vi "Populate VI Help.vi"(5 "API Dir":path[](array[path]), 6 "options":cluster{"Force?(F)":bool, "Show FP":bool}={"Force?(F)"=FALSE, "Show FP"=TRUE}, 7 "doc dir":path, 8 "error in (no error)":errorcluster, 10 "Language Ring":string(combo)="English(en-us)") -> (0 "error out":errorcluster)   [LabVIEW 2017, in "csmdoc.lvlib"]
uses:
  csmdoc.lvlib
  _Typedef/DocElement.ctl
  _Shared/CSM Shared.lvlib
  _tool/_batchEditorDialog/batchEditorDialog.lvlib
  Communicable State Machine.lvlib
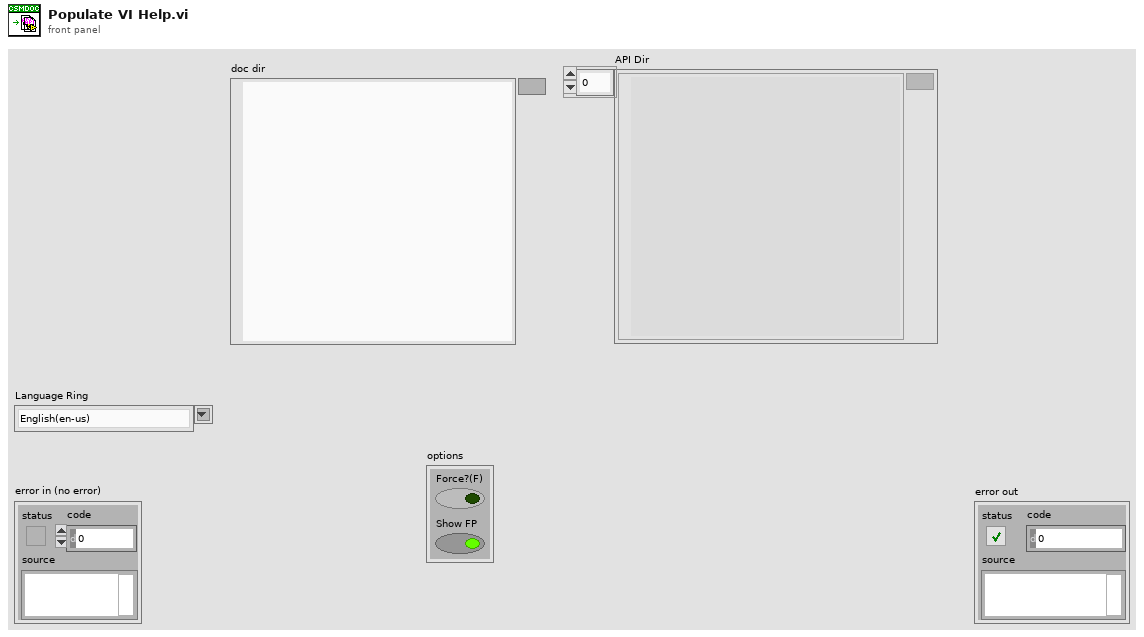
[diagram p1: front panel]
types:
  T1 = typedef "csmdoc.lvlib/DocNote.ctl" = cluster{"ID":string, "Content":string, "Type":string}
  T2 = typedef "csmdoc.lvlib/DocElement.ctl" = cluster{"ID":string, "Content":string[], "SubIDs":string[], "Path":string[]}
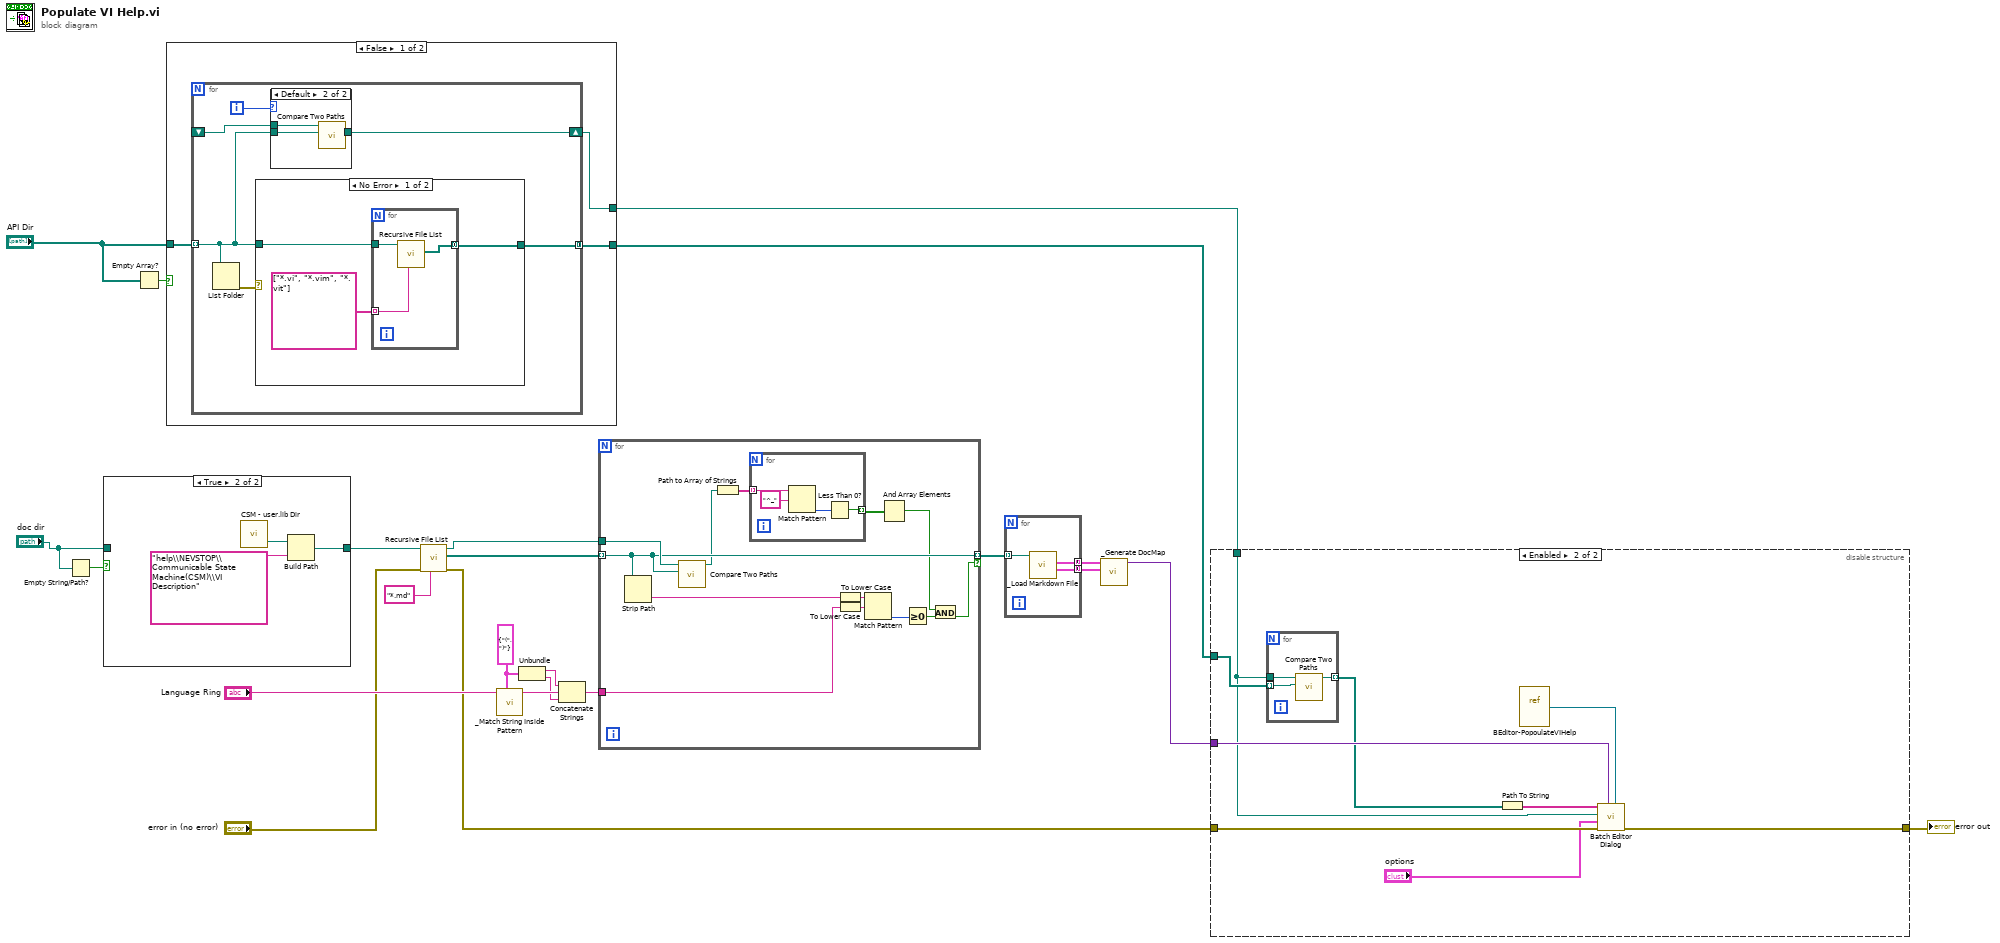
[diagram p0: block diagram]
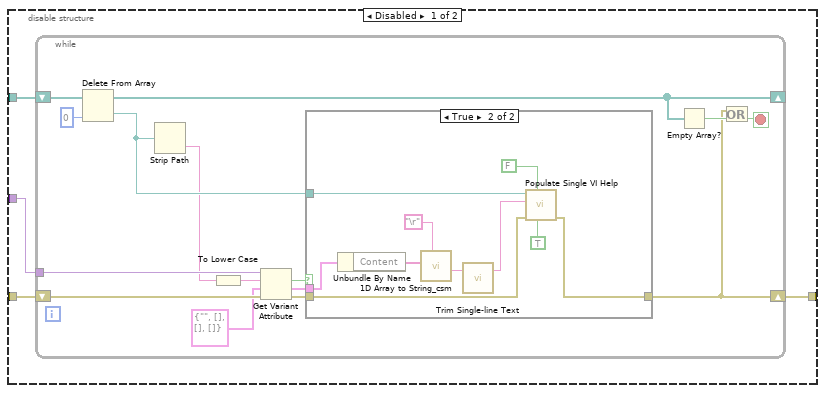
[diagram p2: hidden frame]
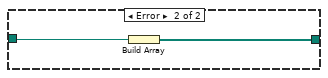
[diagram p5: hidden frame]
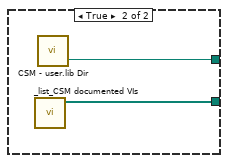
[diagram p6: hidden frame]
diagram:
  w20 = cluster{"left":string, "right":string} {"left"="(", "right"=")"} ("Cluster")
  n1 = Empty String/Path?(string/path="doc dir") -> (empty?=w7:bool)
  n2 = case shown="True" w7 {
    tunnel: [w24 w26] -> w23
    tunnel: "doc dir" -> [w24 _]
    frame False {
    }
    frame True {
      n3 = call "CSM - user.lib Dir.vi"() -> ("<LabVIEW>"=w25:path)  [unwired: 2 in, 1 out]
      n4 = Build Path(base path=w25, name or relative path="help\\NEVSTOP\\Communicable State Machine(CSM)\\VI Description") -> (appended path=w26:path)
    }
  }
  n5 = Empty Array?(array="API Dir") -> (empty?=w5:bool)
  n6 = case shown="False" w5 {
    tunnel: [w30 w50] -> w4
    tunnel: "API Dir" -> [w29 _]
    tunnel: [w28 w49] -> w2
    frame False {
      n7 = for {
        tunnel: [w36] -> w30 mode=concatenating
        tunnel: w29 -> [w32] mode=indexing
        shift-right: [w34] -> w28
        shift-left: _ -> [w33]
        i -> [w31]
        n8 = List Folder(path=w32) -> (error out=w35:errorcluster)  [unwired: 3 in, 3 out]
        n9 = case shown="No Error" w35 {
          tunnel: [w42 w47] -> w36
          tunnel: w32 -> [w41 w48]
          frame No Error {
            n10 = for {
              tunnel: w41 -> [w46]
              tunnel: string[] ["*.vi", "*.vim", "*.vit"] -> [w45] mode=indexing
              tunnel: [w44] -> w42 mode=concatenating
              n11 = call <vilib>:"Recursive File List.vi"("pattern"=w45, "Folder Path"=w46) -> ("All Files in Dir"=w44:path[])  [unwired: 5 in, 4 out]
            }
          }
          frame Error {
            n12 = Build Array(w48) -> (w47:path[])
          }
        }
        n13 = case shown="Default" w31 {
          tunnel: [w37 w40] -> w34
          tunnel: w33 -> [_ w39]
          tunnel: w32 -> [w37 w38]
          frame 0 {
          }
          frame Default {
            n14 = call <vilib>:"Compare Two Paths.vi"("Path 2"=w38, "Path 1"=w39) -> ("Common Path"=w40:path)  [unwired: 6 in, 3 out]
          }
        }
      }
    }
    frame True {
      n15 = call "_list_CSM documented VIs.vi"() -> ("Array"=w50:path[])  [unwired: 11 in]
      n16 = call "CSM - user.lib Dir.vi"() -> ("<LabVIEW>"=w49:path)  [unwired: 2 in, 1 out]
    }
  }
  n17 = call <vilib>:"Recursive File List.vi"("pattern"="*.md", "error in (no error)"="error in (no error)", "Folder Path"=w23) -> ("error out"=w9:errorcluster, "All Files in Dir"=w21:path[], "dup Folder Path"=w1:path)  [unwired: 4 in, 2 out]
  n18 = call "_Match String Inside Pattern.vi"("Cluster"=w20, "string"="Language Ring") -> ("String inside"=w19:string)  [unwired: 8 in, 1 out]
  n19 = Unbundle(w20) -> ("left"=w17:string, "right"=w18:string)
  n20 = Concatenate Strings(w17, w19, w18) -> (w16:string)
  n21 = for {
    tunnel: w21 -> [w56] mode=indexing
    tunnel: [w56] -> w12 mode=indexing if=w52
    tunnel: w16 -> [w62]
    tunnel: w1 -> [w57]
    n22 = Strip Path(path=w56) -> (name=w63:string)  [unwired: 1 out]
    n23 = call <vilib>:"Compare Two Paths.vi"("Path 2"=w56, "Path 1"=w57) -> ("Relative Path from 1 to 2"=w55:path)  [unwired: 6 in, 3 out]
    n24 = Path to Array of Strings(0:w55) -> (2:w54:string[])  [unwired: 1 out]
    n25 = for {
      tunnel: w54 -> [w67] mode=indexing
      tunnel: [w64] -> w53 mode=indexing
      n26 = Match Pattern(string=w67, regular expression="^_") -> (offset past match=w65:i32)  [unwired: 1 in, 3 out]
      n27 = Less Than 0?(x=w65) -> (x < 0?=w64:bool)
    }
    n28 = To Lower Case(string=w63) -> (all lower case string=w58:string)
    n29 = To Lower Case(string=w62) -> (all lower case string=w59:string)
    n30 = Match Pattern(string=w58, regular expression=w59) -> (offset past match=w61:i32)  [unwired: 1 in, 3 out]
    n31 = And Array Elements(Boolean array=w53) -> (logical AND=w51:bool)
    n32 = Greater Or Equal To 0?(x=w61) -> (x >= 0?=w60:bool)
    n33 = And(x=w51, y=w60) -> (x .and. y?=w52:bool)
  }
  n34 = for {
    tunnel: w12 -> [w70] mode=indexing
    tunnel: [w69] -> w14 mode=concatenating
    tunnel: [w68] -> w13 mode=concatenating
    n35 = call "_Load Markdown File.vi"("Path"=w70) -> ("Array 2"=w68:T1[], "Array"=w69:T2[])  [unwired: 8 in, 1 out]
  }
  n36 = call "_Generate DocMap.vi"("Array 2"=w13, "Array"=w14) -> ("Variant"=w8:variant)  [unwired: 9 in]
  n37 = disable-structure shown="Enabled" {
    disable-tunnel: [w74 w108] -> w10
    disable-tunnel: w9 -> [w73 w109]
    disable-tunnel: w8 -> [w72 w107]
    disable-tunnel: w4 -> [w71 w103]
    disable-tunnel: w2 -> [_ w101]
    frame Disabled {
      n38 = while {
        shift-right: [w86] -> _
        shift-left: w71 -> [w88]
        tunnel: w72 -> [w84]
        shift-right: [w75] -> w74
        shift-left: w73 -> [w81]
        stop <- w76 stop-if-true
        n39 = Delete From Array(array=w88, index=0) -> (deleted portion=w89:path, array with subset deleted=w86:path[])  [unwired: 1 in]
        n40 = Strip Path(path=w89) -> (name=w83:string)  [unwired: 1 out]
        n41 = To Lower Case(string=w83) -> (all lower case string=w78:string)
        n42 = Get Variant Attribute(Variant=w84, name=w78, default value (empty Variant)=T2 {"ID"="", "Content"=[], "SubIDs"=[], "Path"=[]} ("Cluster"), error in=w81) -> (found=w82:bool, value=w79:T2, error out=w80:errorcluster)  [unwired: 1 out]
        n43 = case shown="True" w82 {
          tunnel: w89 -> [_ w100]
          tunnel: w80 -> [w90 w99]
          tunnel: [w90 w98] -> w75
          tunnel: w79 -> [_ w94]
          frame False {
          }
          frame True {
            n44 = Unbundle By Name(w94) -> ("Content"=w97:string[])
            n45 = call "1D Array to String_csm.vi"("delimiter (Tab)"="\r", "Array of Strings"=w97) -> ("delimited string"=w95:string)  [unwired: 9 in]
            n46 = call "Trim Single-line Text.vi"("single-line text"=w95) -> ("trimed text"=w93:string)  [unwired: 2 in]
            n47 = call "Populate Single VI Help.vi"("Show FP"=TRUE, "Force?(F)"=FALSE, "error in (no error)"=w99, "VI Description"=w93, "Path"=w100) -> ("error out"=w98:errorcluster)  [unwired: 6 in]
          }
        }
        n48 = Empty Array?(array=w86) -> (empty?=w87:bool)
        n49 = Or(x=w75, y=w87) -> (x .or. y?=w76:bool)
      }
    }
    frame Enabled {
      n50 = for {
        tunnel: w101 -> [w112]
        tunnel: w103 -> [w111] mode=indexing
        tunnel: [w110] -> w102 mode=indexing
        n51 = call <vilib>:"Compare Two Paths.vi"("Path 2"=w111, "Path 1"=w112) -> ("Relative Path from 1 to 2"=w110:path)  [unwired: 6 in, 3 out]
      }
      n52 = Path To String(path=w102) -> (string=w106:string[])
      n53 = vi-ref "BEditor-PopoulateVIHelp.vi"() -> (w105:refnum<vi>)
      n54 = call "Batch Editor Dialog.vi"("VI Refnum"=w105, "Reference"=w107, "Error in"=w109, "Option"="options", "Root"=w101, "Entries"=w106) -> ("Error out"=w108:errorcluster)  [unwired: 5 in]
    }
  }
  "error out" <- w10
